vi "Bai3_5.vi"() -> ()   [LabVIEW 2023]
panel:
  in  "Device Name":tag="Dev8"
  in  "Lines to Write":u16(ring) items=["0 - 7", "8 - 15", "16 - 23"]
  in  "Stop":bool=TRUE
  in  "error in":errorcluster
  out "error out":errorcluster
  in  "stop":bool
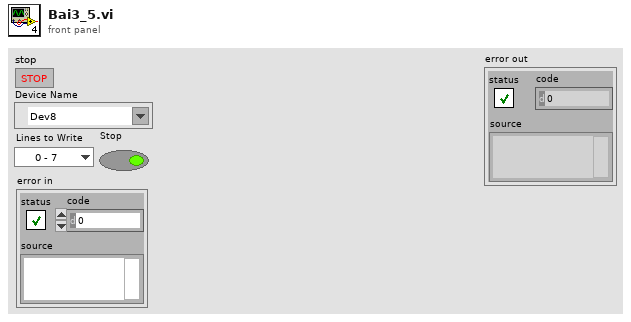
[diagram p1: front panel]
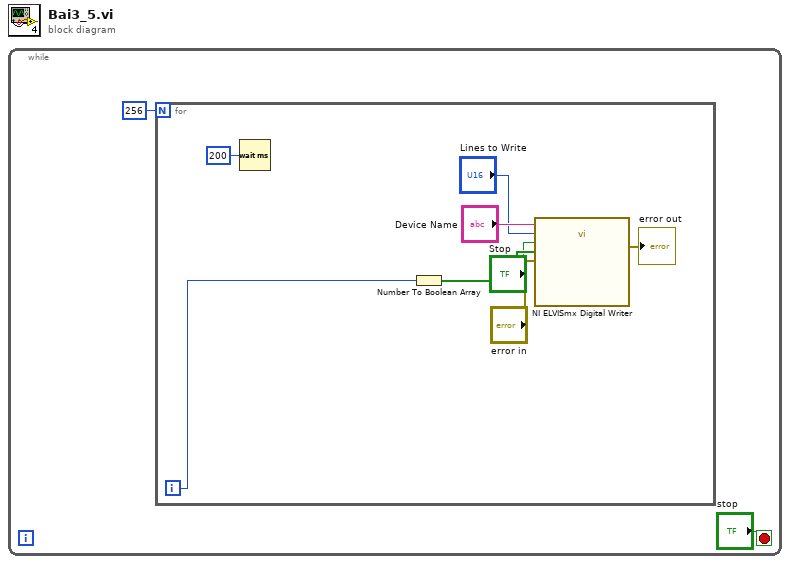
[diagram p0: block diagram]
diagram:
  n1 = while {
    stop <- "stop" stop-if-true
    n2 = for {
      N: 256 -> [_]
      i -> [w3]
      n3 = Wait (ms)(milliseconds to wait=u32 200) -> ()  [unwired: 1 out]
      n4 = Number To Boolean Array(number=w3) -> (Boolean array=w10:bool[])
      n5 = call "NI ELVISmx Digital Writer"("Device Name"="Device Name", "Lines to Write"="Lines to Write", "Stop"="Stop", "DO Lines"=w10, "error in"="error in") -> ("error out"=→"error out":errorcluster)  [unwired: 14 in]
    }
  }
